vi "DatabaseHand_DeleteSubElement.vi"(0 "Database RefNum in":T3, 7 "Object Data In":T1, 9 "Index":i32, 11 "error in (no error)":errorcluster) -> (4 "Database RefNum out":T3, 8 "Object Data Out":T1, 10 "Element deleted":T2, 15 "error out":errorcluster)   [LabVIEW 2016]
doc: "This VI finds the RefNum of an existing object with the input Name or creates a new object if the Name is not found or Name is unwired or an empty string.\nCopyright 2001 VI Engineering, Inc."
uses:
  DatabaseHand_RefNum.ctl
  DatabaseHand_Element.ctl
  DatabaseHan_DatabaseElement.ctl
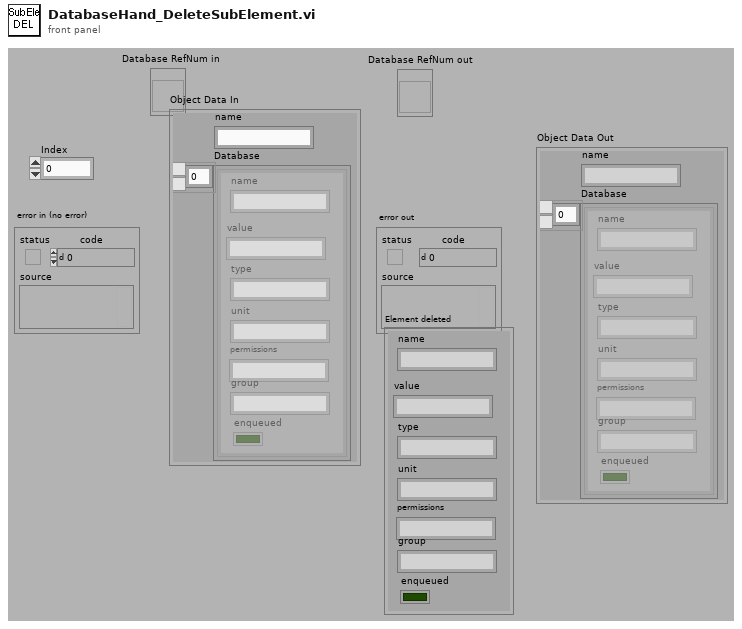
[diagram p1: front panel]
types:
  T1 = typedef "DatabaseHand_Element.ctl" = cluster{"name":string, "Database":T2[]}
  T2 = typedef "DatabaseHan_DatabaseElement.ctl" = cluster{"name":string, "value":string, "type":string, "unit":string, "permissions":string, "enqueued":bool, "group":string}
  T3 = typedef "DatabaseHand_RefNum.ctl" = refnum<vi>
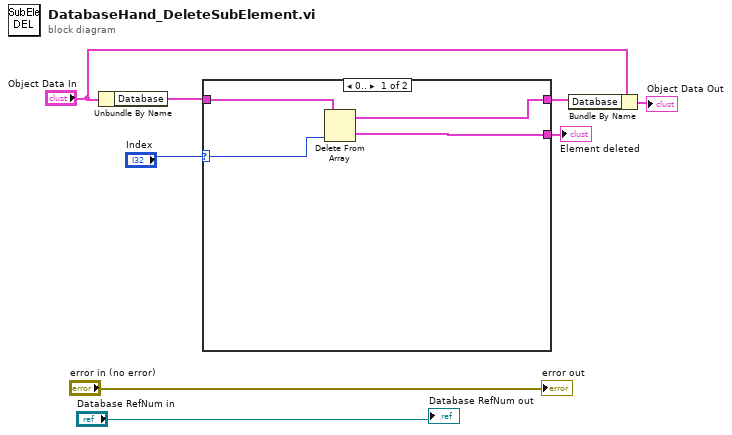
[diagram p0: block diagram]
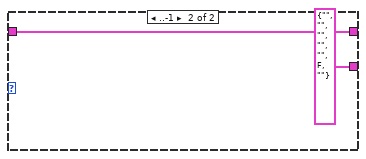
[diagram p2: hidden frame]
diagram:
  n1 = Unbundle By Name("Object Data In") -> ("Database"=w5:T2[])
  n2 = case shown="0.." "Index" {
    selector: "Index" -> [w10 _]
    tunnel: w5 -> [w12 w13]
    tunnel: [w11 T2 {"name"="", "value"="", "type"="", "unit"="", "permissions"="", "enqueued"=FALSE, "group"=""} ("Object Data In")] -> w4
    tunnel: [w9 w13] -> w2
    frame 0.. {
      n3 = Delete From Array(array=w12, index=w10) -> (deleted portion=w11:T2, array with subset deleted=w9:T2[])  [unwired: 1 in]
    }
    frame ..-1 {
    }
  }
  "Element deleted" <- w4
  n4 = Bundle By Name(cluster="Object Data In", "Database"=w2) -> (→"Object Data Out":T1)
  "error out" <- "error in (no error)"
  "Database RefNum out" <- "Database RefNum in"
